vi "Relay Test.vi"() -> ()   [LabVIEW 2012]
uses:
  <vilib>/Rock Robotics/SystemInterfaces/DIO/FPGA_DIORelayChannel.ctl
  <vilib>/Rock Robotics/WPI/Joystick/WPI_JoystickDeviceEnum.ctl
  <vilib>/Rock Robotics/WPI/Relay/WPI_RelayValue.ctl
  <vilib>/Rock Robotics/WPI/Joystick/WPI_JoystickGetSetRefNum.vi
panel:
  in  "Relay B":T1=enum."Relay 8"
  in  "Relay A":T1
  in  "stop":bool
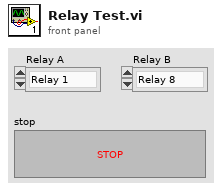
[diagram p1: front panel]
types:
  T1 = typedef "FPGA_DIORelayChannel.ctl" = enum8{"Relay 1", "Relay 2", "Relay 3", "Relay 4", "Relay 5", "Relay 6", "Relay 7", "Relay 8", "Invalid"}
  T2 = typedef "WPI_JoystickDeviceEnum.ctl" = enum16{"USB 1", "USB 2", "USB 3", "USB 4", "Kinect 1", "Kinect 2"}
  T3 = typedef "WPI_JoystickDevRef.ctl" = cluster{"Device":T2}
  T4 = typedef "WPI_RelayValue.ctl" = enum16{"Off", "On", "Forward", "Reverse"}
  T5 = typedef "WPI_RelayDevRef.ctl" = cluster{"DevStatus":errorcluster, "Relay Channel":T1, "Digital Module":T6, "Relay Direction":T7}
  T6 = typedef "FPGA_TypedefDigitalModule.ctl" = enum16{"Digital Module 1", "Digital Module 2"}
  T7 = typedef "WPI_RelayDirection.ctl" = enum16{"Both directions", "Forward only", "Reverse only"}
  T8 = typedef "WPI_JoystickButtonState.ctl" = cluster{"Button 1":bool, "Button 2":bool, "Button 3":bool, "Button 4":bool, "Button 5":bool, "Button 6":bool, "Button 7":bool, "Button 8":bool, "Button 9":bool, "Button 10":bool, "Button 11":bool, "Button 12":bool}
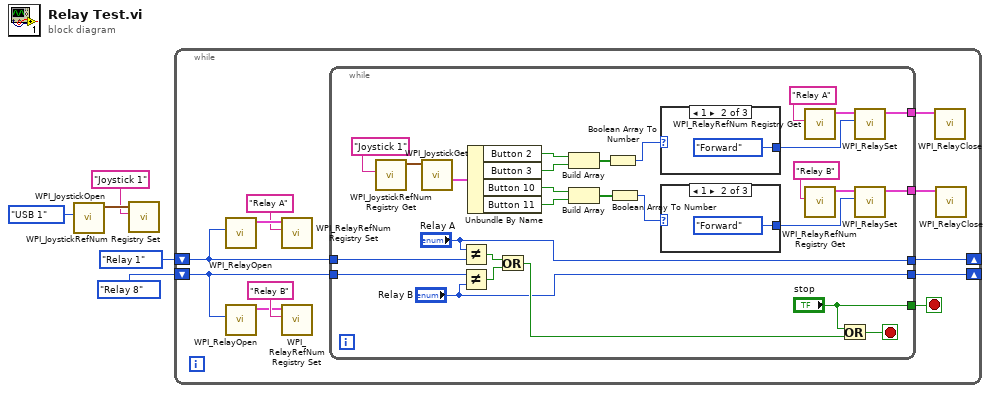
[diagram p0: block diagram]
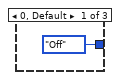
[diagram p2: hidden frame]
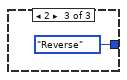
[diagram p3: hidden frame]
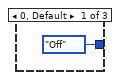
[diagram p4: hidden frame]
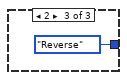
[diagram p5: hidden frame]
diagram:
  n1 = call <vilib>:"WPI_JoystickOpen.vi"("JoystickDevice"=WPI_JoystickDeviceEnum."USB 1") -> ("JoystickDevRef"=w5:T3)  [unwired: 10 in]
  n2 = call <vilib>:"WPI_JoystickRefNum Registry Set.vi"("refnum name"="Joystick 1", "JoystickDevRef"=w5) -> ()  [unwired: 8 in, 2 out]
  n3 = while {
    shift-right: [w9] -> _
    shift-left: FPGA_DIORelayChannel."Relay 1" ("Relay A") -> [w7]
    shift-right: [w8] -> _
    shift-left: FPGA_DIORelayChannel."Relay 8" ("Relay A") -> [w6]
    stop <- w16 stop-if-true
    n4 = call <vilib>:"WPI_RelayOpen.vi"("Relay Channel"=w7) -> ("RelayDevRef"=w15:T5)  [unwired: 9 in, 1 out]
    n5 = call <vilib>:"WPI_RelayOpen.vi"("Relay Channel"=w6) -> ("RelayDevRef"=w12:T5)  [unwired: 9 in, 1 out]
    n6 = call <vilib>:"WPI_RelayRefNum Registry Set.vi"("refnum name"="Relay A", "RelayDevRef"=w15) -> ()  [unwired: 8 in, 2 out]
    n7 = call <vilib>:"WPI_RelayRefNum Registry Set.vi"("refnum name"="Relay B", "RelayDevRef"=w12) -> ()  [unwired: 8 in, 2 out]
    n8 = while {
      tunnel: [w27] -> w11
      tunnel: [w26] -> w10
      tunnel: ["stop"] -> w16
      tunnel: w7 -> [w21]
      tunnel: w6 -> [w20]
      tunnel: ["Relay A"] -> w9
      tunnel: ["Relay B"] -> w8
      stop <- w25 stop-if-true
      n9 = call <vilib>:"WPI_JoystickRefNum Registry Get.vi"("refnum name"="Joystick 1") -> ("JoystickDevRef"=w44:T3)  [unwired: 9 in, 1 out]
      n10 = call <vilib>:"WPI_JoystickGet.vi"("JoystickDevRef"=w44) -> ("Buttons"=w42:T8)  [unwired: 4 in, 2 out]
      n11 = Not Equal?(x="Relay A", y=w21) -> (x != y?=w22:bool)
      n12 = Not Equal?(x=w20, y="Relay B") -> (x != y?=w23:bool)
      n13 = Unbundle By Name(w42) -> ("Button 2"=w41:bool, "Button 3"=w40:bool, "Button 10"=w38:bool, "Button 11"=w39:bool)
      n14 = Or(x=w22, y=w23) -> (x .or. y?=w19:bool)
      n15 = Build Array(w41, w40) -> (w37:bool[])
      n16 = Build Array(w38, w39) -> (w36:bool[])
      n17 = Boolean Array To Number(Boolean array=w37) -> (number=w34:u32)
      n18 = Boolean Array To Number(Boolean array=w36) -> (number=w30:u32)
      n19 = case shown="1" w34 {
        tunnel: [WPI_RelayValue."Off" ("RelayValue") WPI_RelayValue."Forward" ("RelayValue") WPI_RelayValue."Reverse" ("RelayValue")] -> w33
        frame 0, Default {
        }
        frame 1 {
        }
        frame 2 {
        }
      }
      n20 = case shown="1" w30 {
        tunnel: [WPI_RelayValue."Off" ("RelayValue") WPI_RelayValue."Forward" ("RelayValue") WPI_RelayValue."Reverse" ("RelayValue")] -> w32
        frame 0, Default {
        }
        frame 1 {
        }
        frame 2 {
        }
      }
      n21 = call <vilib>:"WPI_RelayRefNum Registry Get.vi"("refnum name"="Relay A") -> ("RelayDevRef"=w35:T5)  [unwired: 9 in, 1 out]
      n22 = call <vilib>:"WPI_RelayRefNum Registry Get.vi"("refnum name"="Relay B") -> ("RelayDevRef"=w31:T5)  [unwired: 9 in, 1 out]
      n23 = Or(x="stop", y=w19) -> (x .or. y?=w25:bool)
      n24 = call <vilib>:"WPI_RelaySet.vi"("RelayValue"=w33, "RelayDevRef"=w35) -> ("RelayDevRef"=w27:T5)  [unwired: 8 in, 1 out]
      n25 = call <vilib>:"WPI_RelaySet.vi"("RelayValue"=w32, "RelayDevRef"=w31) -> ("RelayDevRef"=w26:T5)  [unwired: 8 in, 1 out]
    }
    n26 = call <vilib>:"WPI_RelayClose.vi"("RelayDevRef"=w11) -> ()  [unwired: 10 in, 1 out]
    n27 = call <vilib>:"WPI_RelayClose.vi"("RelayDevRef"=w10) -> ()  [unwired: 10 in, 1 out]
  }
